vi "FV-calculate_values.vi"(9 "S11_Imag":dbl[](array[numeric]), 10 "S11_Real":dbl[](array[numeric]), 11 "Frequency":dbl[](array[numeric])) -> (1 "complex":T4, 2 "Calc":T3, 3 "Raw":T1)   [LabVIEW 2020, in "FV-file_viewer.lvlib"]
uses:
  FV-file_viewer.lvlib
  FV-complex_cluster.ctl
  FV-single_complex_XY_plot.ctl
  FV-calc_cluster.ctl
  FV-single_XY_plot.ctl
  FV-raw_cluster.ctl
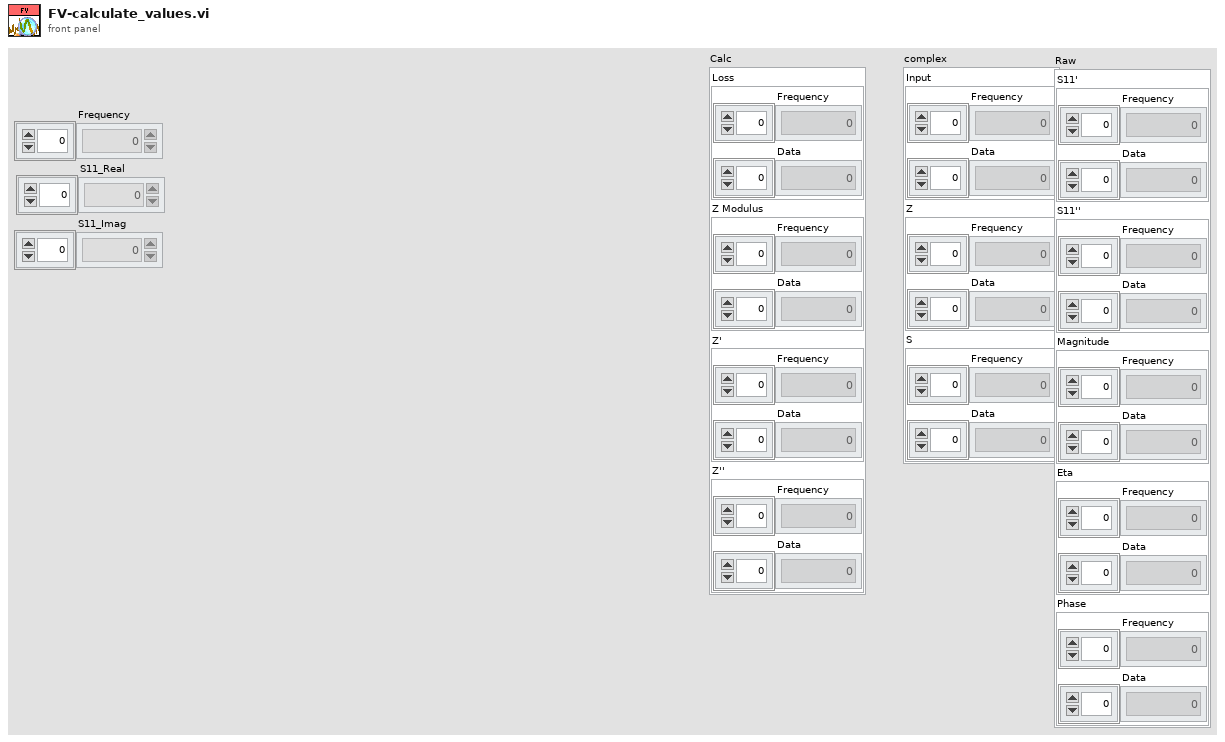
[diagram p1: front panel]
types:
  T1 = typedef "FV-file_viewer.lvlib/FV-raw_cluster.ctl" = cluster{"S11'":T2, "S11''":T2, "Magnitude":T2, "Eta":T2, "Phase":T2}
  T2 = typedef "FV-file_viewer.lvlib/FV-single_XY_plot.ctl" = cluster{"Frequency":dbl[], "Data":dbl[]}
  T3 = typedef "FV-file_viewer.lvlib/FV-calc_cluster.ctl" = cluster{"Loss":T2, "Z Modulus":T2, "Z'":T2, "Z''":T2}
  T4 = typedef "FV-file_viewer.lvlib/FV-complex_cluster.ctl" = cluster{"Input":T5, "Z":T5, "S":T5}
  T5 = typedef "FV-file_viewer.lvlib/FV-single_complex_XY_plot.ctl" = cluster{"Frequency":dbl[], "Data":cdb[]}
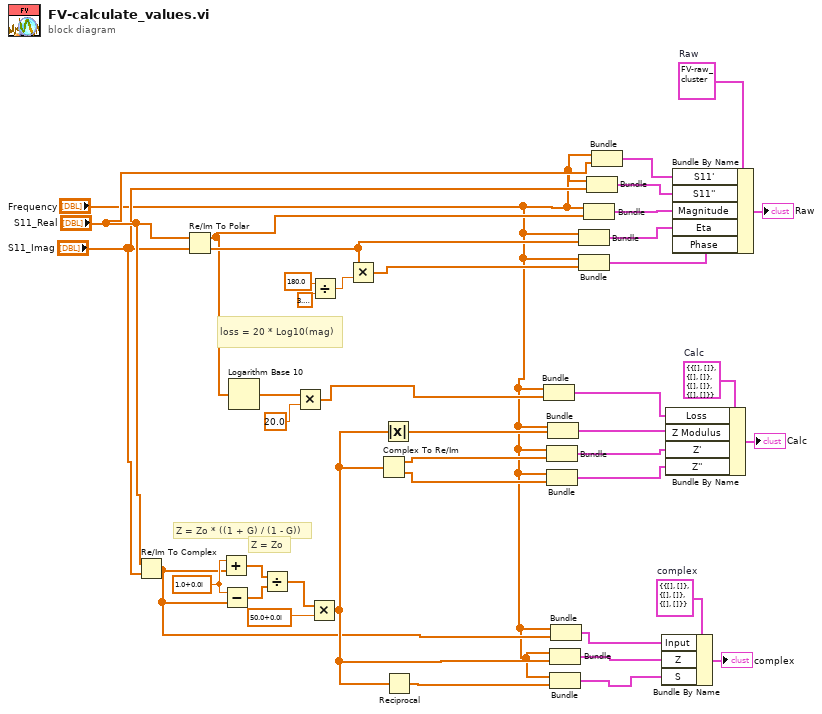
[diagram p0: block diagram]
diagram:
  w6 = T4 {"Input"={"Frequency"=[], "Data"=[]}, "Z"={"Frequency"=[], "Data"=[]}, "S"={"Frequency"=[], "Data"=[]}}  # complex
  w4 = T3 {"Loss"={"Frequency"=[], "Data"=[]}, "Z Modulus"={"Frequency"=[], "Data"=[]}, "Z'"={"Frequency"=[], "Data"=[]}, "Z''"={"Frequency"=[], "Data"=[]}}  # Calc
  w2 = T1 {"S11'"={"Frequency"=[], "Data"=[]}, "S11''"={"Frequency"=[], "Data"=[]}, "Magnitude"={"Frequency"=[], "Data"=[]}, "Eta"={"Frequency"=[], "Data"=[]}, "Phase"={"Frequency"=[], "Data"=[]}}  # Raw
  w36 = cdb 1.0+0.0i ("x")
  # "Z = Zo"
  # "Z = Zo * ((1 + G) / (1 - G))"
  # "loss = 20 * Log10(mag)"
  n1 = Re/Im To Complex(1:"S11_Imag", 2:"S11_Real") -> (0:w22:cdb[])
  n2 = Re/Im To Polar(2:"S11_Imag", 3:"S11_Real") -> (0:w30:dbl[], 1:w24:dbl[])
  n3 = Add(x=w36, y=w22) -> (x+y=w35:cdb[])
  n4 = Subtract(x=w36, y=w22) -> (x-y=w34:cdb[])
  n5 = Logarithm Base 10(1:w24) -> (0:w38:dbl[])
  n6 = Divide(x=w35, y=w34) -> (x/y=w33:cdb[])
  n7 = Multiply(x=w38, y=20.0) -> (x*y=w28:dbl[])
  n8 = Multiply(x=w33, y=cdb 50.0+0.0i) -> (x*y=w23:cdb[])
  n9 = Divide(x=180.0, y=3.141592653589793) -> (x/y=w39:dbl)
  n10 = Multiply(x=w30, y=w39) -> (x*y=w29:dbl[])
  n11 = Complex To Re/Im(x + iy=w23) -> (x=w26:dbl[], y=w25:dbl[])
  n12 = Absolute Value(x=w23) -> (abs(x)=w27:dbl[])
  n13 = Reciprocal(x=w23) -> (1/x=w31:cdb[])
  n14 = Bundle("Frequency"="Frequency", w28) -> (w14:cluster{"Frequency":dbl[], dbl[]})  [unwired: 1 in]
  n15 = Bundle("Frequency"="Frequency", w26) -> (w12:cluster{"Frequency":dbl[], dbl[]})  [unwired: 1 in]
  n16 = Bundle("Frequency"="Frequency", w25) -> (w11:cluster{"Frequency":dbl[], dbl[]})  [unwired: 1 in]
  n17 = Bundle("Frequency"="Frequency", w27) -> (w13:cluster{"Frequency":dbl[], dbl[]})  [unwired: 1 in]
  n18 = Bundle("Frequency"="Frequency", w23) -> (w9:cluster{"Frequency":dbl[], cdb[]})  [unwired: 1 in]
  n19 = Bundle("Frequency"="Frequency", w31) -> (w8:cluster{"Frequency":dbl[], cdb[]})  [unwired: 1 in]
  n20 = Bundle("Frequency"="Frequency", w22) -> (w10:cluster{"Frequency":dbl[], cdb[]})  [unwired: 1 in]
  n21 = Bundle("Frequency"="Frequency", w30) -> (w16:cluster{"Frequency":dbl[], dbl[]})  [unwired: 1 in]
  n22 = Bundle("Frequency"="Frequency", w29) -> (w15:cluster{"Frequency":dbl[], dbl[]})  [unwired: 1 in]
  n23 = Bundle("Frequency"="Frequency", w24) -> (w17:cluster{"Frequency":dbl[], dbl[]})  [unwired: 1 in]
  n24 = Bundle("Frequency"="Frequency", "S11_Imag"="S11_Imag") -> (w18:cluster{"Frequency":dbl[], "S11_Imag":dbl[]})  [unwired: 1 in]
  n25 = Bundle("Frequency"="Frequency", "S11_Real"="S11_Real") -> (w19:cluster{"Frequency":dbl[], "S11_Real":dbl[]})  [unwired: 1 in]
  n26 = Bundle By Name(cluster=w6, "Input"=w10, "Z"=w9, "S"=w8) -> (→"complex":T4)
  n27 = Bundle By Name(cluster=w4, "Loss"=w14, "Z Modulus"=w13, "Z'"=w12, "Z''"=w11) -> (→"Calc":T3)
  n28 = Bundle By Name(cluster=w2, "S11'"=w19, "S11''"=w18, "Magnitude"=w17, "Eta"=w16, "Phase"=w15) -> (→"Raw":T1)
